vi "Out_S10F2.vi"(8 "error in (no error)":errorcluster, 10 "S10F2":T1, 11 "S10 Message Class in":refnum<class "S10 Message Class.lvclass">) -> (0 "error out":errorcluster, 3 "S10 Message Class out":refnum<class "S10 Message Class.lvclass">)   [LabVIEW 2020, in "SECS Communication.lvlib" / "S10 Message Class.lvclass"]
uses:
  S10 Message Class.lvclass
  D:/Dropbox/SECS/LabVIEW Code/Com/SECS Communication/SECS-II Class/SECS-II Class.lvclass
  S10F2.ctl
  SECS-II Class/Data Message_Binary.vi
  S10 Message Class.lvclass/S10 Message Class.ctl
  SECS-II Class/SECS-II Class.lvclass
  D:/Dropbox/SECS/LabVIEW Code/Com/SECS Communication/S10 Message Class/S10 Message Class.lvclass
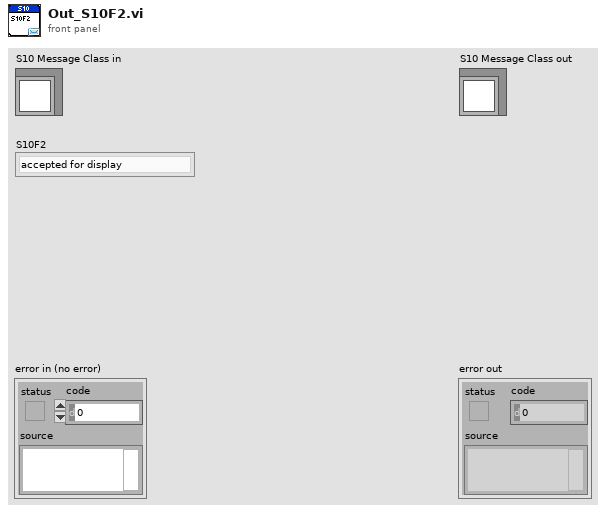
[diagram p1: front panel]
types:
  T1 = typedef "SECS Communication.lvlib/S10 Message Class.lvclass/S10F2.ctl" = enum8{"accepted for display", "message will not be displayed", "terminal not available"}
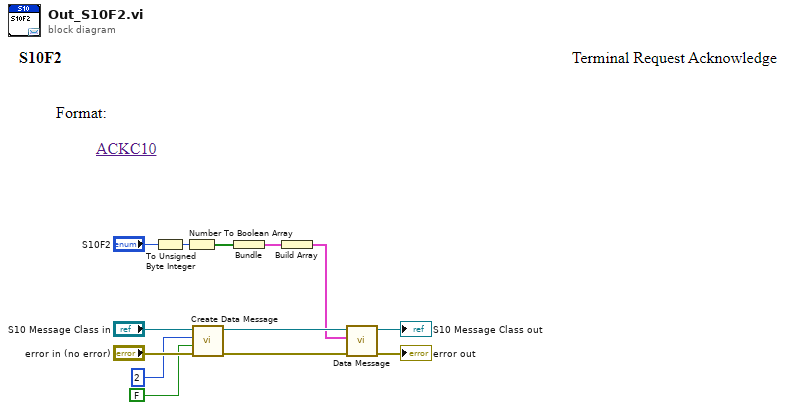
[diagram p0: block diagram]
diagram:
  n1 = To Unsigned Byte Integer(number="S10F2") -> (unsigned 8bit integer=w4:u8)
  n2 = Number To Boolean Array(number=w4) -> (Boolean array=w7:bool[])
  n3 = call "Create Data Message.vi"("error in (no error)"="error in (no error)", "W-Bit"=FALSE, "Function"=u8 2, "SECS-II Class in"="S10 Message Class in") -> ("error out"=w12:errorcluster, "SECS-II Class out"=w13:refnum<class "S10 Message Class.lvclass">)  [unwired: 6 in]
  n4 = Bundle("Boolean array"=w7) -> (w6:cluster{"Boolean array":bool[]})  [unwired: 1 in]
  n5 = Build Array(w6) -> (w3:cluster{"Boolean array":bool[]}[])
  n6 = call-poly "Data Message.vi"("error in"=w12, "Data Cluster"=w3, "SECS-II Class in"=w13) -> ("error out"=→"error out":errorcluster, "SECS-II Class out"=→"S10 Message Class out":refnum<class "S10 Message Class.lvclass">)  [unwired: 7 in]
